vi "DisableMultiple.vi"(6 "return immediately":bool, 8 "error in (no error)":errorcluster, 9 "taskId":i32(ring) items=["TLibrary", "T01", "T02", "T03", "T04", "T05", "T06", "T07", "T08", "T09", "T10", "T11", "T12", "T13", "T14", "T15", "T16", "T17", "T18", "T19", "T20", "T21", "T22", "T23", "T24", "T25", "T26", "T27", "T28", "T29", "T30", "T31"], 10 "axis names":string[](array[string])=["X", "Y"], 11 "controller in":refnum<k24>) -> (0 "error out":errorcluster, 3 "controller out":refnum<k24>)   [LabVIEW 2016]
uses:
  C:/Users/sciollalab/Documents/Brandeis-BNL/LabVIEW_Codes/BNL_ThermomechanicalStave/AerotechLibraries/Bin/Aerotech.A3200.dll
  Bin/Aerotech.A3200.dll
  C:/Users/sciollalab/Documents/Brandeis-BNL/LabVIEW_Codes/BNL_ThermomechanicalStave/AerotechLibraries/Bin/Aerotech.A3200.LabVIEW.dll
  Bin/Aerotech.A3200.LabVIEW.dll
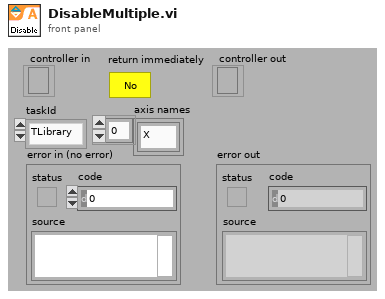
[diagram p1: front panel]
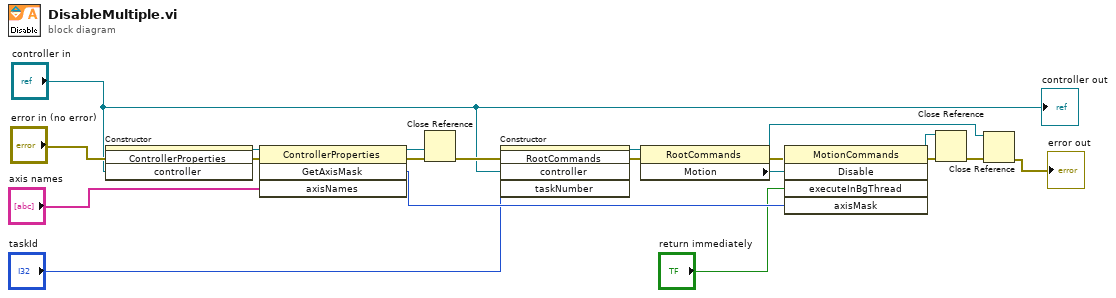
[diagram p0: block diagram]
diagram:
  n1 = constructor class="ControllerProperties"(error in="error in (no error)", "controller"="controller in") -> (reference out=w19:refnum<k24>, error out=w18:errorcluster)  [unwired: 2 in, 2 out]
  n2 = invoke class="ControllerProperties" method="GetAxisMask"(reference=w19, error in=w18, "axisNames"="axis names") -> (reference out=w16:refnum<k24>, error out=w17:errorcluster, "GetAxisMask"=w15:i32)  [unwired: 1 in, 1 out]
  n3 = Close Reference(reference=w16, error in (no error)=w17) -> (error out=w11:errorcluster)
  n4 = constructor class="RootCommands"(error in=w11, "controller"="controller in", "taskNumber"="taskId") -> (reference out=w7:refnum<k24>, error out=w6:errorcluster)  [unwired: 2 in, 3 out]
  n5 = property class="RootCommands"(reference=w7, error in=w6) -> (reference out=w2:refnum<k24>, error out=w8:errorcluster, "Motion"=w9:refnum<k24>)
  n6 = invoke class="MotionCommands" method="Disable"(reference=w9, error in=w8, "executeInBgThread"="return immediately", "axisMask"=w15) -> (reference out=w4:refnum<k24>, error out=w5:errorcluster)  [unwired: 1 in, 3 out]
  n7 = Close Reference(reference=w4, error in (no error)=w5) -> (error out=w3:errorcluster)
  n8 = Close Reference(reference=w2, error in (no error)=w3) -> (error out=→"error out":errorcluster)
  "controller out" <- "controller in"
